vi "SetDarkOffsetCancel.vi"(3 "resource name":string="USB0::0x1313::0x8078::P0005368::INSTR") -> (0 "error out":errorcluster {"code" format="%.0x"})   [LabVIEW 2015]
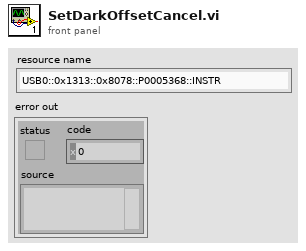
[diagram p1: front panel]
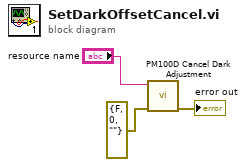
[diagram p0: block diagram]
diagram:
  n1 = call "PM100D Cancel Dark Adjustment.vi"("error in (no error)"=errorcluster {"status"=FALSE, "code"=0, "source"=""}, "instrument handle"="resource name") -> ("error out"=→"error out":errorcluster)  [unwired: 8 in, 1 out]
